vi "PROJEKT.vi"() -> ()   [LabVIEW 2020]
uses:
  <vilib>/Instr/_visa.llb/VISA Configure Serial Port (Instr).vi
panel:
  in  "VISA resource name":refnum<visa-resource-name>="COM5"
  out "String":string
  out "serial monitor":string
  in  "Sampling Time (ms)":dbl=100.0
  in  "stop":bool
  in  "Set point":dbl(slide) scale=0.0..100.0
  in  "Kd":dbl
  in  "Ki":dbl
  in  "Kp":dbl
  in  "baud rate (9600)":u32=9600
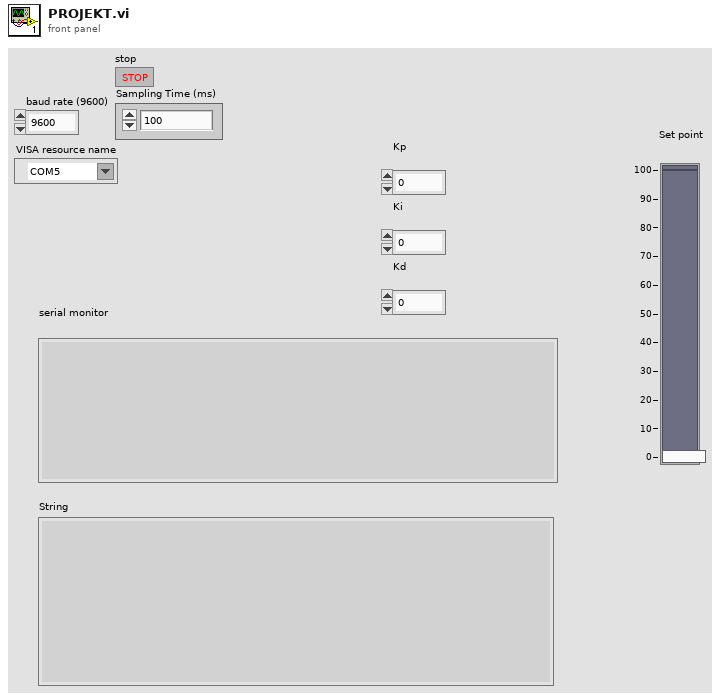
[diagram p1: front panel]
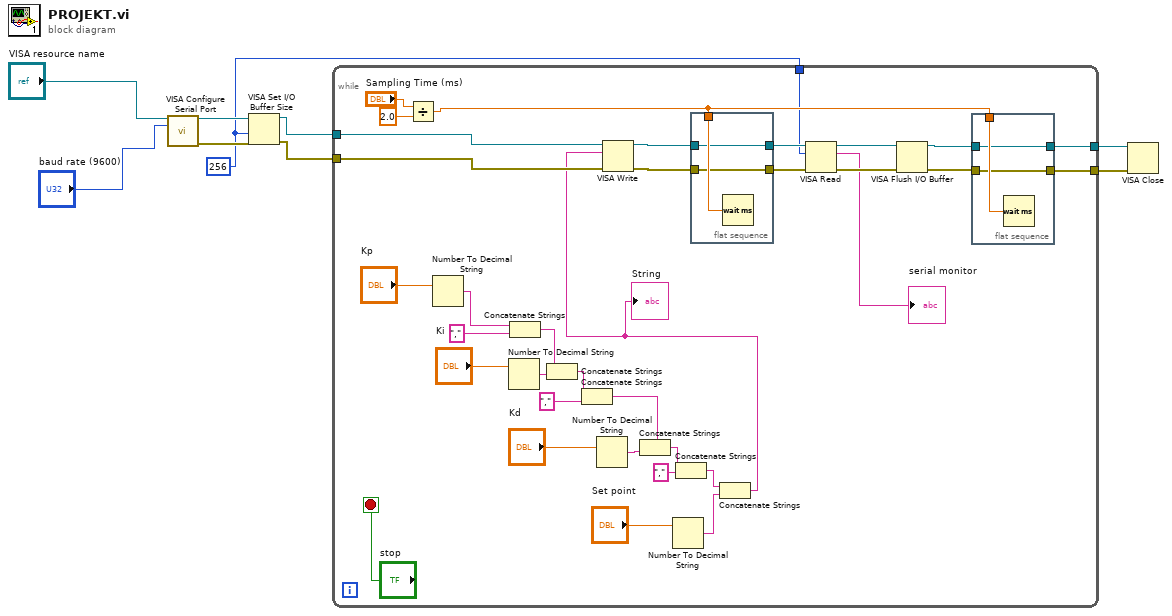
[diagram p0: block diagram]
diagram:
  w2 = u32 256 ("size (4096)")
  n1 = call-poly "VISA Configure Serial Port"("VISA resource name"="VISA resource name", "baud rate (9600)"="baud rate (9600)") -> ("VISA resource name out"=w8:refnum<visa-resource-name>, "error out"=w7:errorcluster)  [unwired: 12 in]
  n2 = VISA Set I/O Buffer Size(VISA resource name=w8, size (4096)=w2, error in (no error)=w7) -> (VISA resource name out=w6:refnum<visa-resource-name>, error out=w5:errorcluster)  [unwired: 1 in]
  n3 = while {
    tunnel: w6 -> [w27]
    tunnel: w5 -> [w26]
    tunnel: [w14] -> w4
    tunnel: [w13] -> w3
    tunnel: w2 -> [w12]
    stop <- "stop" stop-if-true
    n4 = Divide(x="Sampling Time (ms)", y=2.0) -> (x/y=w17:dbl)
    n5 = Number To Decimal String(number="Kp") -> (decimal integer string=w39:string)  [unwired: 1 in]
    n6 = Number To Decimal String(number="Ki") -> (decimal integer string=w36:string)  [unwired: 1 in]
    n7 = Concatenate Strings(w39, ",") -> (w37:string)
    n8 = Concatenate Strings(w37, w36) -> (w35:string)
    n9 = Concatenate Strings(w35, ",") -> (w33:string)
    n10 = Number To Decimal String(number="Kd") -> (decimal integer string=w32:string)  [unwired: 1 in]
    n11 = Concatenate Strings(w33, w32) -> (w31:string)
    n12 = Number To Decimal String(number="Set point") -> (decimal integer string=w28:string)  [unwired: 1 in]
    n13 = Concatenate Strings(w31, ",") -> (w29:string)
    n14 = flat-sequence {
      tunnel: w17 -> [w50]
      tunnel: [w49] -> w20
      tunnel: w22 -> [w49]
      tunnel: [w48] -> w21
      tunnel: w23 -> [w48]
      frame #0 {
        n15 = Wait (ms)(milliseconds to wait=w50) -> ()  [unwired: 1 out]
      }
    }
    n16 = Concatenate Strings(w29, w28) -> (w10:string)
    "String" <- w10
    n17 = VISA Write(VISA resource name=w27, write buffer=w10, error in (no error)=w26) -> (VISA resource name out=w23:refnum<visa-resource-name>, error out=w22:errorcluster)  [unwired: 1 out]
    n18 = VISA Read(VISA resource name=w21, byte count=w12, error in (no error)=w20) -> (VISA resource name out=w19:refnum<visa-resource-name>, read buffer=→"serial monitor":string, error out=w18:errorcluster)  [unwired: 1 out]
    n19 = VISA Flush I/O Buffer(VISA resource name=w19, error in (no error)=w18) -> (VISA resource name out=w16:refnum<visa-resource-name>, error out=w15:errorcluster)  [unwired: 1 in]
    n20 = flat-sequence {
      tunnel: w17 -> [w47]
      tunnel: [w46] -> w13
      tunnel: w15 -> [w46]
      tunnel: [w45] -> w14
      tunnel: w16 -> [w45]
      frame #0 {
        n21 = Wait (ms)(milliseconds to wait=w47) -> ()  [unwired: 1 out]
      }
    }
  }
  n22 = VISA Close(VISA resource name=w4, error in (no error)=w3) -> ()  [unwired: 1 out]
